vi "LIN Write.vi"(5 "Len":u32, 6 "Data":u8[](array[numeric])=[0, 0, 0, 0, 0, 0, 0, 0, 0], 7 "DataLen":u8, 9 "ID":u8, 10 "LINIndex":u8, 11 "DevHandle":i32) -> (3 "function return":i32)   [LabVIEW 2010, in "usb2lin.lvlib"]
doc: "int WINAPI LIN_Write(int DevHandle,unsigned char LINIndex,LIN_MSG *pLINMsg,unsigned int Len);"
uses:
  usb2lin.lvlib
  USB2XXX/trunk/USB2XXX/USB2XXX/vs2010/Release/USB2XXX.dll
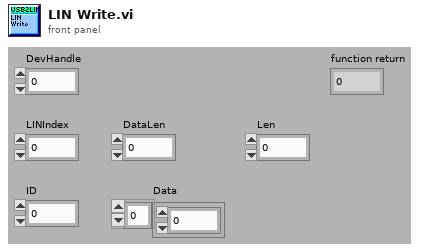
[diagram p1: front panel]
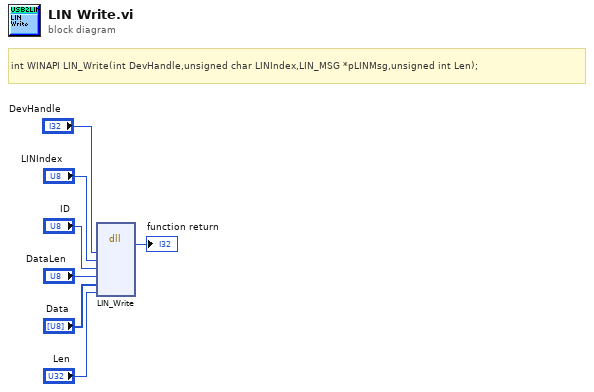
[diagram p0: block diagram]
diagram:
  # "int WINAPI LIN_Write(int DevHandle,unsigned char LINIndex,LIN_MSG *pLINMsg,unsigned int Len);"
  n1 = dll-call lib="E:/OtherWork/STM32/USB2XXX/trunk/USB2XXX/USB2XXX/vs2010/Release/USB2XXX.*" fn="LIN_Write"("DevHandle"="DevHandle", "LINIndex"="LINIndex", "ID"="ID", "DataLen"="DataLen", "Data"="Data", "Len"="Len") -> (→"function return":i32)  [unwired: 9 in, 2 out]
